vi "W&R(Know Size Compare Check WithOut Data).vi"(0 "VISA resource name in":refnum<visa-resource-name>, 5 "写入指令/数据":string, 7 "比较校验":string, 9 "超时":u32=5000, 11 "error in":errorcluster) -> (4 "VISA resource name out":refnum<visa-resource-name>, 6 "布尔":bool, 8 "码词":string, 15 "error out":errorcluster)   [LabVIEW 2020]
uses:
  <vilib>/Instr/_visa.llb/VISA Flush IO Buffer Mask.ctl
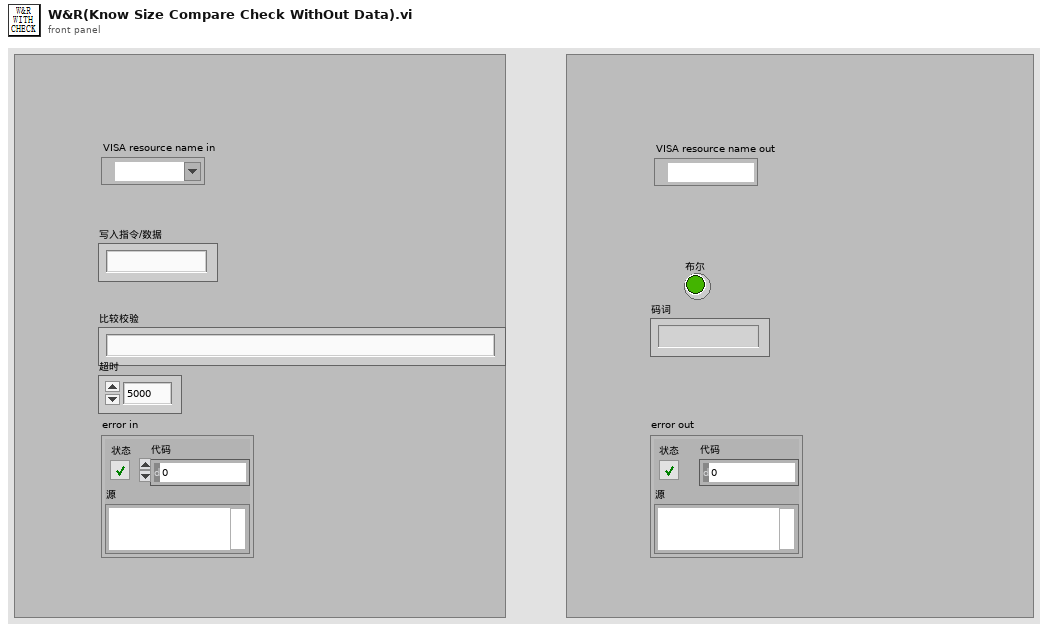
[diagram p1: front panel]
types:
  T1 = typedef "VISA Flush IO Buffer Mask.ctl" = u16
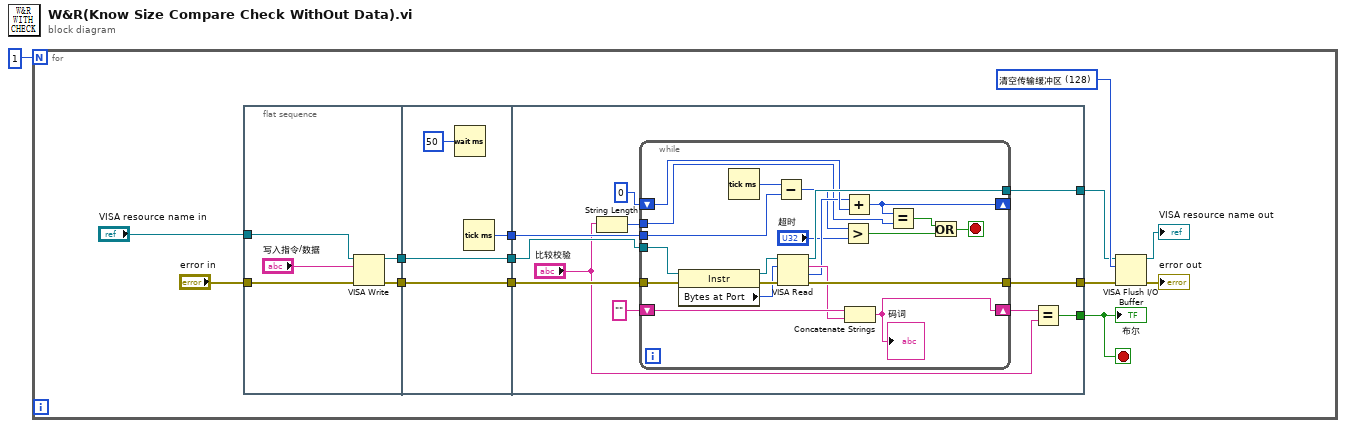
[diagram p0: block diagram]
diagram:
  n1 = for {
    N: 1 -> [_]
    stop <- w2 stop-if-true
    w7 = T1 128 items=["清空接收缓冲区"=16, "向设备写入传输缓冲区"=32, "清空接收缓冲区（无I/O）"=64, "清空传输缓冲区"=128] ("Mask")
    n2 = flat-sequence {
      tunnel: "VISA resource name in" -> [w19]
      tunnel: [w18] -> w14
      tunnel: [w16] -> w13
      tunnel: "error in" -> [w15]
      tunnel: [w23] -> w12
      tunnel: w14 -> [w23]
      tunnel: [w22] -> w11
      tunnel: w13 -> [w22]
      tunnel: [w21] -> w10
      tunnel: w12 -> [w34]
      tunnel: w11 -> [w33]
      tunnel: [w24] -> w2
      tunnel: [w32] -> w6
      tunnel: [w31] -> w4
      tunnel: w10 -> [w28]
      frame #0 {
        n3 = VISA Write(VISA resource name=w19, write buffer="写入指令/数据", error in (no error)=w15) -> (VISA resource name out=w18:refnum<visa-resource-name>, error out=w16:errorcluster)  [unwired: 1 out]
      }
      frame #1 {
        n4 = Wait (ms)(milliseconds to wait=u32 50 ("等待时间（毫秒）")) -> ()  [unwired: 1 out]
        n5 = Tick Count (ms)() -> (millisecond timer value=w21:u32)
      }
      frame #2 {
        n6 = String Length(string="比较校验") -> (length=w27:i32)
        n7 = while {
          tunnel: w34 -> [w55]
          tunnel: w33 -> [w54]
          shift-right: [w51] -> w25
          shift-left: "" -> [w50]
          tunnel: [w49] -> w32
          tunnel: [w48] -> w31
          shift-right: [w44] -> _
          shift-left: u32 0 -> [w45]
          tunnel: w28 -> [w41]
          tunnel: w27 -> [w35]
          stop <- w37 stop-if-true
          n8 = property class="Instr"(reference=w55, error in=w54) -> (reference out=w53:refnum<visa-resource-name>, error out=w52:errorcluster, "Bytes at Port"=w46:u32)
          n9 = Tick Count (ms)() -> (millisecond timer value=w42:u32)
          n10 = Subtract(x=w42, y=w41) -> (x-y=w40:u32)
          n11 = VISA Read(VISA resource name=w53, byte count=w46, error in (no error)=w52) -> (VISA resource name out=w49:refnum<visa-resource-name>, read buffer=w47:string, return count=w43:u32, error out=w48:errorcluster)
          n12 = Greater?(x=w40, y="超时") -> (0:w38:bool)
          n13 = Add(x=w43, y=w45) -> (x+y=w44:u32)
          n14 = Concatenate Strings(w50, w47) -> (w51:string)
          "码词" <- w51
          n15 = Equal?(x=w44, y=w35) -> (x = y?=w39:bool)
          n16 = Or(x=w39, y=w38) -> (x .or. y?=w37:bool)
        }
        n17 = Equal?(x=w25, y="比较校验") -> (x = y?=w24:bool)
      }
    }
    n18 = VISA Flush I/O Buffer(VISA resource name=w6, mask (16)=w7, error in (no error)=w4) -> (VISA resource name out=→"VISA resource name out":refnum<visa-resource-name>, error out=→"error out":errorcluster)
    "布尔" <- w2
  }
